vi "PECT_GateConverse.vi"(9 "Gate 2":dbl=25.0, 10 "Gate 1":dbl, 11 "Freq_Sampling_SizeX_SizeY":dbl[](array[numeric])) -> (0 "Length T/2":i32, 1 "Length":i32, 2 "Start 2":i32, 3 "Start 1":i32, 4 "Length T":i32)   [LabVIEW 2018]
panel:
  # "%"
  # "%"
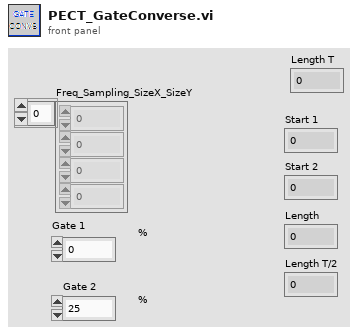
[diagram p1: front panel]
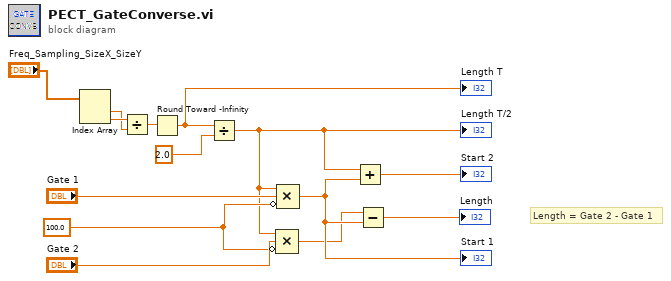
[diagram p0: block diagram]
diagram:
  w10 = 100.0 ("蔼")
  # "Length = Gate 2 - Gate 1"
  n1 = Index Array(array="Freq_Sampling_SizeX_SizeY") -> (element #1=w4:dbl, element #2=w5:dbl)  [unwired: 2 in]
  n2 = Divide(x=w5, y=w4) -> (x/y=w7:dbl)
  n3 = Round Toward -Infinity(1:w7) -> (0:w1:dbl)
  "Length T" <- w1
  n4 = Divide(x=w1, y=2.0) -> (x/y=w8:dbl)
  "Length T/2" <- w8
  n5 = Compound Arithmetic op=MULTIPLY(w8, "Gate 2", invert w10) -> (w9:dbl)
  n6 = Compound Arithmetic op=MULTIPLY(w8, "Gate 1", invert w10) -> (w12:dbl)
  "Start 1" <- w12
  n7 = Add(x=w8, y=w12) -> (x+y=→"Start 2":dbl)
  n8 = Subtract(x=w9, y=w12) -> (x-y=→"Length":dbl)
